vi "TEST - MD5 Hash.vi"(8 "error in (no error)":errorcluster) -> (0 "error out":errorcluster, 2 "Pass":bool)   [LabVIEW 2009]
panel:
  out "Failures":T1(array[cluster])
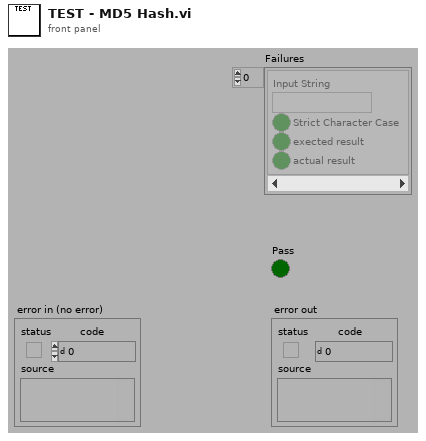
[diagram p1: front panel]
types:
  T1 = cluster{"Input String":string, "Strict Character Case":bool, "exected result":bool, "actual result":bool}[]
  T2 = cluster{"Input String":string, "Strict Character Case":bool, "Expected Result":bool, "Actual Result":bool}[]
  T3 = cluster{"Input String":string, "Strict Character Case":bool, "Expected Result":bool, "Actual Result":bool}
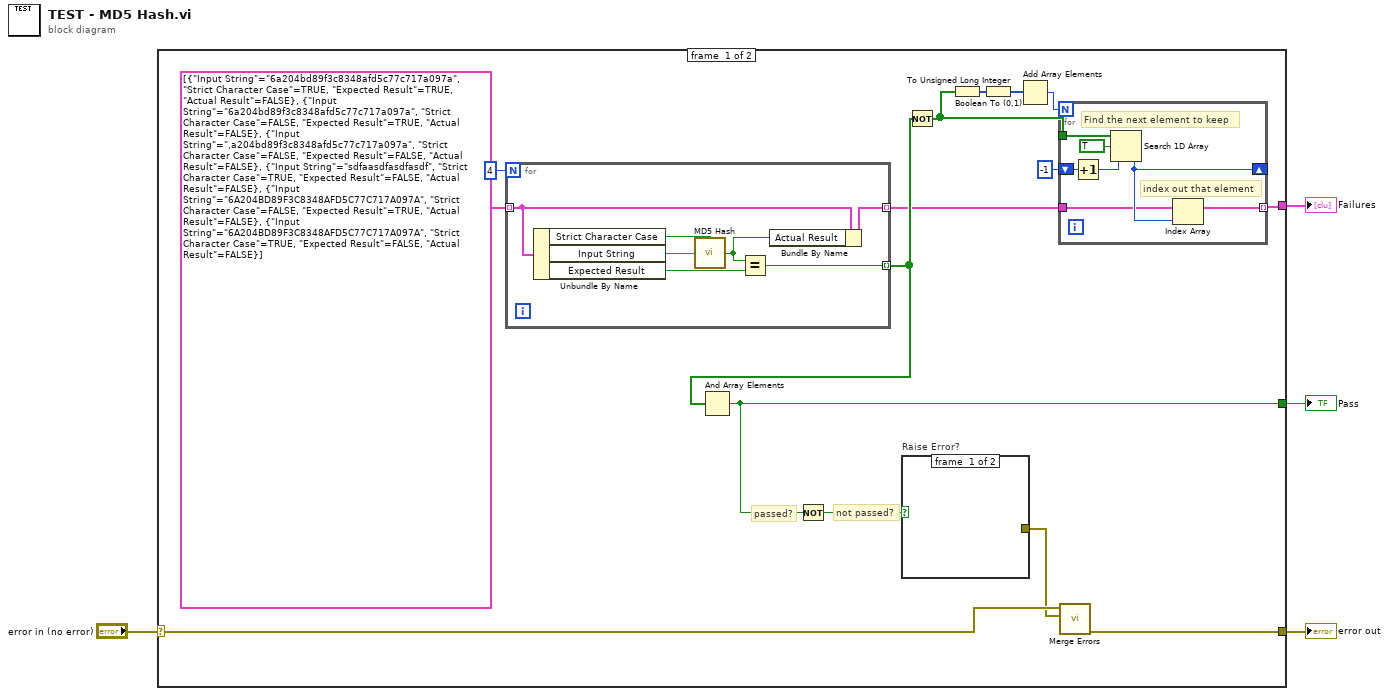
[diagram p0: block diagram]
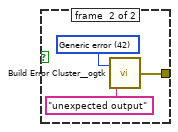
[diagram p2: hidden frame]
diagram:
  n1 = case shown="No Error" "error in (no error)" {
    selector: "error in (no error)" -> [w19 w37]
    tunnel: [w14 _] -> w4
    tunnel: [w18 w37] -> w2
    tunnel: [w6 _] -> w1
    frame #0 {
      # "not passed?"
      # "passed?"
      n2 = for {
        N: 4 -> [_]
        tunnel: T2 [{"Input String"="6a204bd89f3c8348afd5c77c717a097a", "Strict Character Case"=TRUE, "Expected Result"=TRUE, "Actual Result"=FALSE}, {"Input String"="6a204bd89f3c8348afd5c77c717a097a", "Strict Character Case"=FALSE, "Expected Result"=TRUE, "Actual Result"=FALSE}, {"Input String"=",a204bd89f3c8348afd5c77c717a097a", "Strict Character Case"=FALSE, "Expected Result"=FALSE, "Actual Result"=FALSE}, {"Input String"="sdfaasdfasdfasdf", "Strict Character Case"=TRUE, "Expected Result"=FALSE, "Actual Result"=FALSE}, {"Input String"="6A204BD89F3C8348AFD5C77C717A097A", "Strict Character Case"=FALSE, "Expected Result"=TRUE, "Actual Result"=FALSE}, {"Input String"="6A204BD89F3C8348AFD5C77C717A097A", "Strict Character Case"=TRUE, "Expected Result"=FALSE, "Actual Result"=FALSE}] -> [w30] mode=indexing
        tunnel: [w33] -> w8 mode=indexing
        tunnel: [w31] -> w7 mode=indexing
        n3 = Unbundle By Name(w30) -> ("Strict Character Case"=w27:bool, "Input String"=w29:string, "Expected Result"=w32:bool)
        n4 = call "MD5 Hash.vi"("Strict Case? (False)"=w27, "Input String"=w29) -> ("MD5 Hash?"=w28:bool)  [unwired: 2 in]
        n5 = Equal?(x=w28, y=w32) -> (x = y?=w33:bool)
        n6 = Bundle By Name(cluster=w30, "Actual Result"=w28) -> (w31:T3)
      }
      n7 = And Array Elements(Boolean array=w8) -> (logical AND=w14:bool)
      n8 = Not(x=w14) -> (.not. x?=w16:bool)
      n9 = case "Raise Error?" shown="True" w16 {
        tunnel: [_ w34] -> w17
        frame #0 {
        }
        frame #1 {
          w35 = 42 items=["No error", "Argument error", "Memory is full", "Out of zone", "End of file", "File already open", "Generic file I/O error", "File not found", "File permission error", "Disk is full", "Duplicate path", "Too many files open", "System feature not enabled", "Resource file not found", "Cannot add resource", "Resource not found", "Image not found", "Image memory error", "Pen does not exist", "Config type invalid", "Config token not found", "Config parse error", "Config memory error", "Bad external code format", "Bad external code offset", "External code not present", "Null window", "Destroy window error", "Null menu", "Print aborted", "Bad print record", "Print driver error", "Windows error during printing", "Memory error during printing", "Print dialog error", "Generic print error", "Invalid device refnum", "Device not found", "Device parameter error", "Device unit error", "Cannot open device", "Device call aborted", "Generic error", "Cancelled by user", "Object ID too low", "Object ID too high", "Object not in heap", "Unknown heap", "Unknown object (invalid DefProc)", "Unknown object (DefProc not in table)", "Message out of range", "Invalid (null) method", "Unknown message", "Manager call not supported", "Bad address", "Network operation in progress", "Network operation timed out", "Connection is busy", "Network attribute not supported", "Network error", "Address in use", "System out of memory", "Connection aborted", "Connection refused", "Not connected", "Already connected", "Connection closed", "Initialization error (interapplication manager)", "Bad occurrence", "Wait on unbound occurrence handler", "Occurrence queue overflow", "Datalog type conflict", "Unused", "Unrecognized type (interapplication manager)", "Memory corrupt", "Failed to make temporary DLL", "Old CIN version", "Drag socket not found", "Failed to load drop-object", "Failed to register OLE object", "Failed to release OLE object", "Format specifier type mismatch", "Unknown format specifier", "Too few format specifiers", "Too many format specifiers", "Scan failed", "Newer CIN version", "Error converting to variant", "Runtime menu error", "Password tampered", "Variant attribute not found", "Incompatible variant data type", "Event data is not available", "Event Store is not present", "Occurrence is not found", "Event Queue is not created", "Event info is not available", "Refnum passed is NULL", "Error retrieving Class GUID", "Error retrieving CoClass GUID", "Error retrieving TypeLib GUID.", "Bad built application magic bytes.", "Specific driver is different from the specific driver associated with the Logical Name.", "There is no session opened to the class driver.", "Max Error", "MAX - Error with config objects", "MAX - Error loading configuration", "MAX - Group not supported"]
          n10 = call <userlib>:"Build Error Cluster__ogtk.vi"("String to Prepend to source (\"\")"="unexpected output" ("String to Prepend to source (\"\")"), "code"=w35) -> ("error out"=w34:errorcluster)
        }
      }
      n11 = Not(x=w8) -> (.not. x?=w10:bool[])
      n12 = Boolean To (0,1)(Boolean=w10) -> (0, 1=w11:i16[])
      n13 = To Unsigned Long Integer(number=w11) -> (unsigned 32bit integer=w9:u32[])
      n14 = Add Array Elements(numeric array=w9) -> (sum=w12:u32)
      n15 = for {
        N: w12 -> [_]
        tunnel: w7 -> [w22]
        tunnel: w10 -> [w26]
        shift-right: [w23] -> _
        shift-left: -1 ("start index (0)") -> [w24]
        tunnel: [w21] -> w6 mode=indexing
        # "index out that element"
        # "Find the next element to keep"
        n16 = Increment(x=w24) -> (x+1=w20:i32)
        n17 = Search 1D Array(1D array=w26, element=TRUE, start index (0)=w20) -> (index of element=w23:i32)
        n18 = Index Array(array=w22, index=w23) -> (element=w21:T3)
      }
      n19 = call <vilib>:"Merge Errors.vi"("error in 2 (no error)"=w17, "error in 1 (no error)"=w19) -> ("error out"=w18:errorcluster)  [unwired: 5 in]
    }
    frame #1 {
    }
  }
  "Pass" <- w4
  "error out" <- w2
  "Failures" <- w1
